vi "code rev.vi"() -> (0 "Found Revision":bool, 3 "Code Revision":string)   [LabVIEW 2014]
uses:
  <vilib>/Rock Robotics/Network Tables/NT Read String.vi
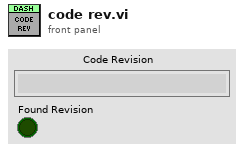
[diagram p1: front panel]
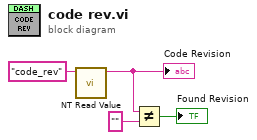
[diagram p0: block diagram]
diagram:
  n1 = call-poly <vilib>:"NT Read Value.vi"("Name"="code_rev") -> ("String"=w3:string)  [unwired: 9 in, 1 out]
  "Code Revision" <- w3
  n2 = Not Equal?(x=w3, y="") -> (x != y?=→"Found Revision":bool)
